vi "Track Goals VP.vi"(0 "Image In":T2, 7 "error in":errorcluster) -> (20 "Image Out":T2, 26 "Target Report (calibrated)":T1(array[cluster]) {"Score" format="%.2f"; "Centroid"."y" format="%.2f"; "Centroid"."x" format="%.2f"}, 27 "error out":errorcluster)   [LabVIEW 2015]
uses:
  <vilib>/vision/Image Controls.llb/IMAQ Image.ctl
  <vilib>/vision/NI_Vision_Development_Module.lvlib
panel:
  out "Target Report (raw)":T1(array[cluster]) {"Score" format="%.2f"; "Centroid"."y" format="%.2f"; "Centroid"."x" format="%.2f"}
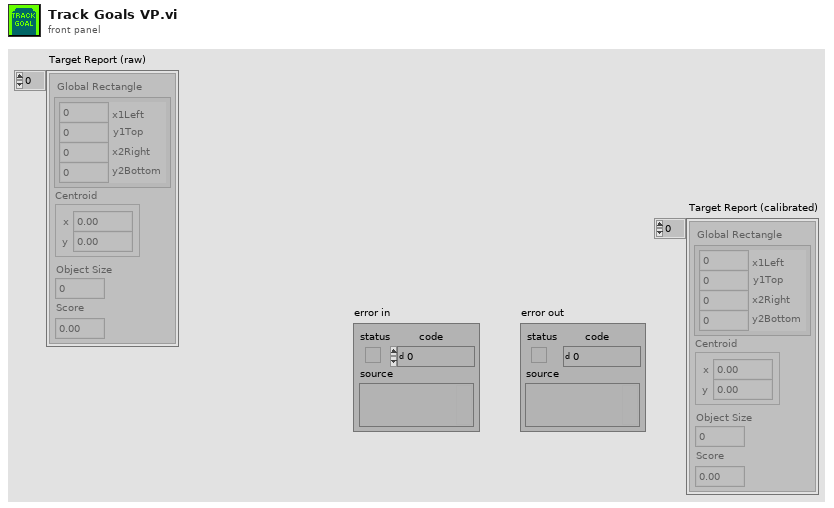
[diagram p1: front panel]
types:
  T1 = cluster{"Global Rectangle":cluster{"x1Left":i32, "y1Top":i32, "x2Right":i32, "y2Bottom":i32}, "Centroid":cluster{"x":sgl, "y":sgl}, "Object Size":u32, "Score":dbl}[]
  T2 = typedef "IMAQ Image.ctl" = refnum<image>
  T3 = cluster{"Brightness":sgl, "Contrast":sgl, "Gamma":sgl}
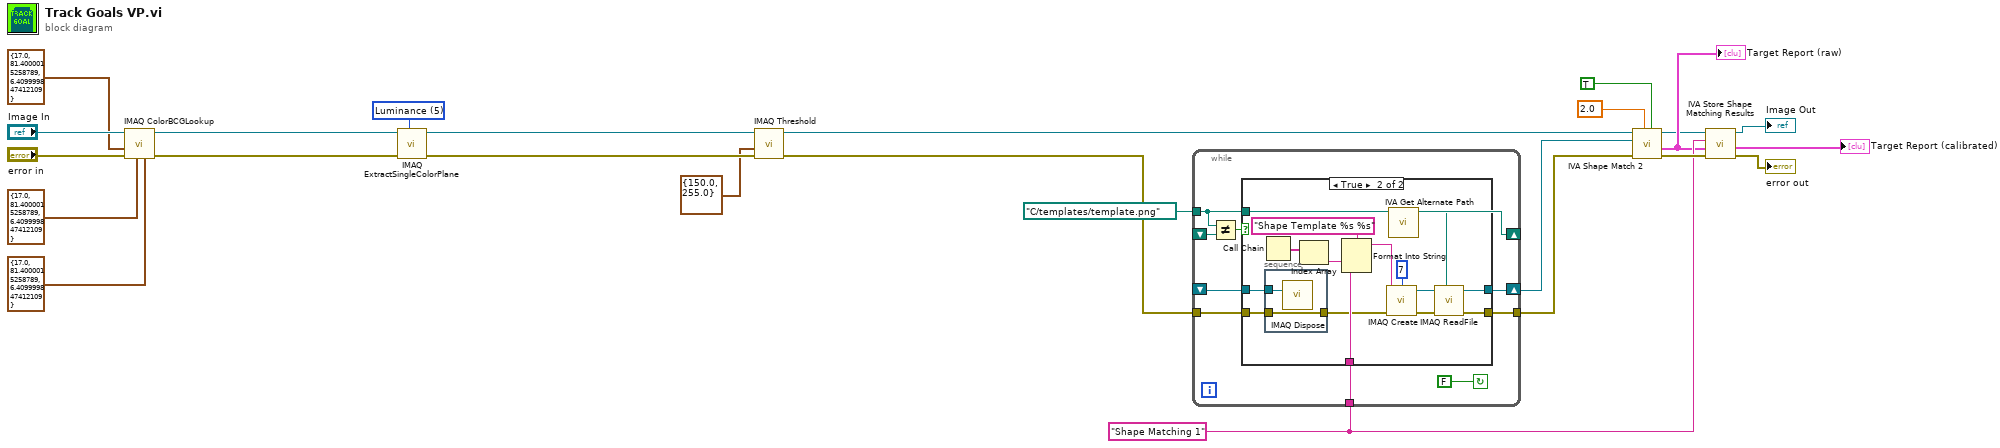
[diagram p0: block diagram]
diagram:
  w7 = "Shape Matching 1" ("Step Name")
  w19 = 5 items=["Red", "Green", "Blue", "Hue", "Saturation", "Luminance", "Value", "Intensity"] ("Color Plane")
  n1 = call "IMAQ ColorBCGLookup"("Blue BCG Values"=T3 {"Brightness"=17.0, "Contrast"=81.4, "Gamma"=6.41}, "Green BCG Values"=T3 {"Brightness"=17.0, "Contrast"=81.4, "Gamma"=6.41}, "error in (no error)"="error in", "Red BCG Values"=T3 {"Brightness"=17.0, "Contrast"=81.4, "Gamma"=6.41}, "Image Src"="Image In") -> ("error out"=w23:errorcluster, "Image Dst Out"=w18:T2)  [unwired: 2 in, 3 out]
  n2 = call "IMAQ ExtractSingleColorPlane"("Color Plane"=w19, "error in (no error)"=w23, "Image Src"=w18) -> ("error out"=w17:errorcluster, "Image Dst Out"=w15:T2)  [unwired: 1 in, 6 out]
  n3 = call "IMAQ Threshold"("error in (no error)"=w17, "Range"=cluster{"Lower value":sgl, "Upper value":sgl} {"Lower value"=150.0, "Upper value"=255.0}, "Image Src"=w15) -> ("error out"=w14:errorcluster, "Image Dst Out"=w5:T2)  [unwired: 3 in, 4 out]
  n4 = while {
    shift-right: [w34] -> w4
    shift-left: _ -> [w33]
    tunnel: [w31] -> w8
    tunnel: w14 -> [w30]
    tunnel: path "C:/templates/template.png" ("Template Path") -> [w28]
    tunnel: w7 -> [w29]
    shift-right: [w28] -> _
    shift-left: _ -> [w27]
    stop <- FALSE continue-if-true
    n5 = Not Equal?(x=w28, y=w27) -> (x != y?=w26:bool)
    n6 = case shown="True" w26 {
      tunnel: [w36 w48] -> w34
      tunnel: w33 -> [w36 w39]
      tunnel: [w35 w46] -> w31
      tunnel: w30 -> [w35 w38]
      tunnel: w28 -> [_ w41]
      tunnel: w29 -> [_ w42]
      frame False {
      }
      frame True {
        n7 = Call Chain() -> (call chain=w44:string[])
        n8 = stacked-sequence {
          tunnel: w39 -> [w53]
          tunnel: w38 -> [w52]
          tunnel: [w52] -> w37
          frame #0 {
            n9 = call "IMAQ Dispose"("Image"=w53) -> ()  [unwired: 2 in, 4 out]
          }
        }
        n10 = Index Array(array=w44) -> (element=w43:string)  [unwired: 1 in]
        n11 = Format Into String(format string="Shape Template %s %s" ("Image Name"), w43, w42) -> (resulting string=w51:string)  [unwired: 2 in, 1 out]
        n12 = call "IMAQ Create"("Border Size"=7, "Image Name"=w51, "error in (no error)"=w37) -> ("New Image"=w49:T2, "error out"=w47:errorcluster)  [unwired: 1 in, 1 out]
        n13 = call <vilib>:"IVA Get Alternate Path.vi"("Path In"=w41) -> ("Path Out"=w40:path)  [unwired: 10 out]
        n14 = call "IMAQ ReadFile"("File Path"=w40, "error in (no error)"=w47, "Image"=w49) -> ("error out"=w46:errorcluster, "Image Out"=w48:T2)  [unwired: 2 in, 5 out]
      }
    }
  }
  n15 = call <vilib>:"IVA Shape Match 2.vi"("Scale Invariance"=TRUE, "Minimal Score"=2.0, "error in (no error)"=w8, "Template"=w4, "Image Src"=w5) -> ("error out"=w11:errorcluster, "Shape Report"=w3:T1, "Image Out"=w2:T2)  [unwired: 4 out]
  "Target Report (raw)" <- w3
  n16 = call <vilib>:"IVA Store Shape Matching Results.vi"("error in (no error)"=w11, "Shape Report"=w3, "Step Name"=w7, "Image in"=w2) -> ("error out"=→"error out":errorcluster, "Shape Report (calibrated)"=→"Target Report (calibrated)":T1, "Image dup"=→"Image Out":T2)  [unwired: 5 out]
